vi "Kicker - Wait Unil Ready.vi"(8 "error in (no error)":errorcluster) -> (0 "error out":errorcluster)   [LabVIEW 2015]
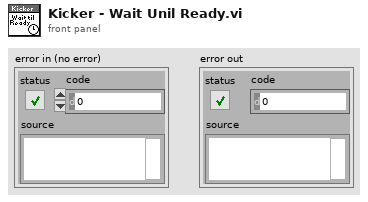
[diagram p1: front panel]
types:
  T1 = typedef "WPI_SwitchDevRef.ctl" = cluster{"DevStatus":errorcluster, "DIO Channel":T2, "CntIndex":T3, "Normally Closed":bool}
  T2 = typedef "FPGA_DIOChannel.ctl" = enum8{"DIO 0", "DIO 1", "DIO 2", "DIO 3", "DIO 4", "DIO 5", "DIO 6", "DIO 7", "DIO 8", "DIO 9", "DIO MXP 0", "DIO MXP 1", "DIO MXP 2", "DIO MXP 3", "DIO MXP 4", "DIO MXP 5", "DIO MXP 6", "DIO MXP 7", "DIO MXP 8", "DIO MXP 9", "DIO MXP 10", "DIO MXP 11", "DIO MXP 12", "DIO MXP 13", "DIO MXP 14", "DIO MXP 15", "Invalid"}
  T3 = typedef "FPGA_CounterCtrSystemIndex.ctl" = enum8{"Ctr 0", "Ctr 1", "Ctr 2", "Ctr 3", "Ctr 4", "Ctr 5", "Ctr 6", "Ctr 7", "Invalid"}
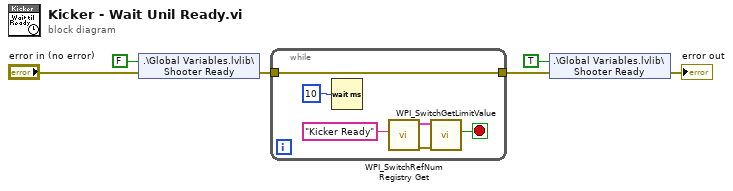
[diagram p0: block diagram]
diagram:
  n1 = shared-variable ".\\Global Variables.lvlib\\Shooter Ready"(FALSE ("Shooter Ready"), error in="error in (no error)") -> (error out=w4:errorcluster)
  n2 = while {
    tunnel: [w7] -> w3
    tunnel: w4 -> [w7]
    stop <- w10 stop-if-true
    n3 = Wait (ms)(milliseconds to wait=u32 10) -> ()  [unwired: 1 out]
    n4 = call <vilib>:"WPI_SwitchRefNum Registry Get.vi"("refnum name"="Kicker Ready") -> ("error out"=w11:errorcluster, "SwitchDevRef"=w9:T1)  [unwired: 9 in]
    n5 = call <vilib>:"WPI_SwitchGetLimitValue.vi"("error in (no error)"=w11, "SwitchDevRef"=w9) -> ("Switch Pressed"=w10:bool)  [unwired: 7 in, 2 out]
  }
  n6 = shared-variable ".\\Global Variables.lvlib\\Shooter Ready"(TRUE ("Shooter Ready"), error in=w3) -> (error out=→"error out":errorcluster)
